vi "Read Init Cricket.vi"(8 "error in (no error)":errorcluster, 11 "Cricket in":refnum<class "Cricket.lvclass">) -> (0 "error out":errorcluster, 2 "Init Cricket":timestamp, 3 "Cricket out":refnum<class "Cricket.lvclass">)   [LabVIEW 2021, in "Cricket.lvclass"]
uses:
  Cricket.lvclass
  Cricket.lvclass/Cricket.ctl
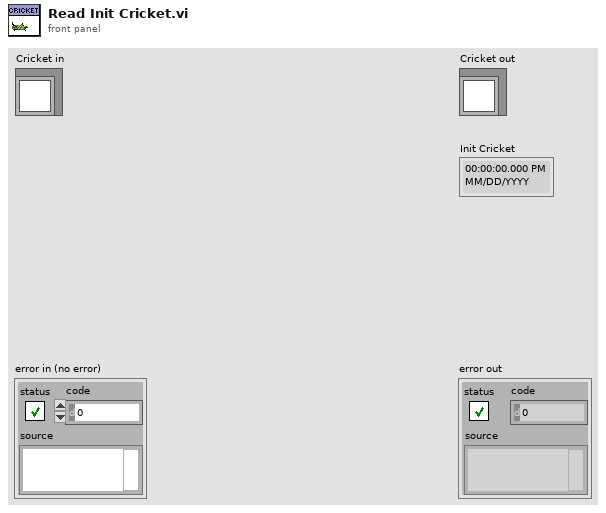
[diagram p1: front panel]
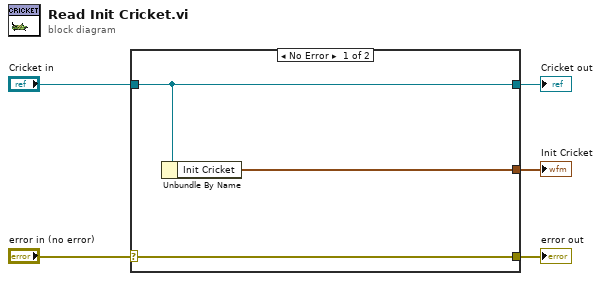
[diagram p0: block diagram]
diagram:
  n1 = case shown="No Error" "error in (no error)" {
    selector: "error in (no error)" -> [w8 w9]
    tunnel: [w8 w9] -> w4
    tunnel: [w7 w10] -> w2
    tunnel: "Cricket in" -> [w7 w10]
    tunnel: [w6 _] -> w1
    frame No Error {
      n2 = Unbundle By Name(w7) -> ("Init Cricket"=w6:timestamp)
    }
    frame Error {
    }
  }
  "error out" <- w4
  "Cricket out" <- w2
  "Init Cricket" <- w1
